vi "Aquire LMS Data.vi"(10 "LMS Information Cluster In":T2) -> (2 "LMS Information Cluster Out":T1)   [LabVIEW 2014]
uses:
  Hokuyo URG Series.lvlib
panel:
  in  "Number of Scans":dbl
  in  "Scan Interval":dbl
  in  "Encoding Width":u16(ring)=3 items=["2 Byte"=2, "3 Byte"=3]
  in  "Cluster Count":dbl=1.0
  in  "Start Point":dbl=-135.0
  in  "End Point":dbl=135.0
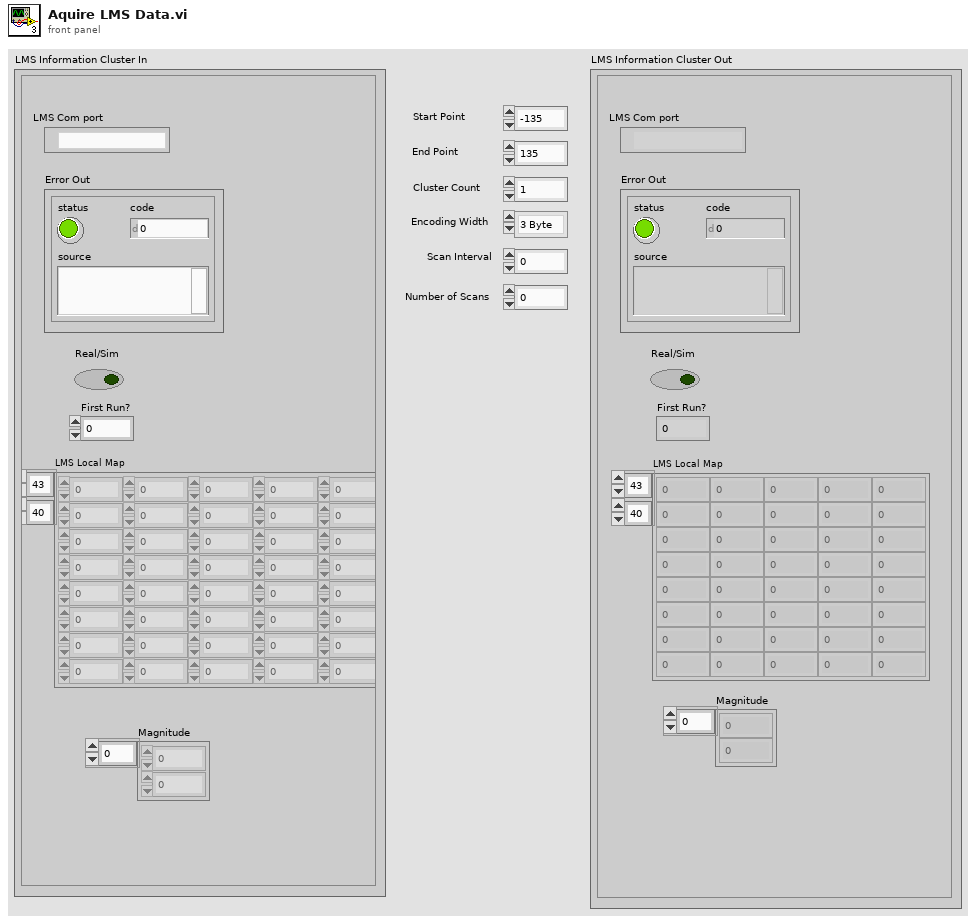
[diagram p1: front panel]
types:
  T1 = cluster{"LMS Com port":refnum<visa-resource-name>, "Error Out":errorcluster, "Real/Sim":bool, "First Run?":i32, "LMS Local Map ":dbl[][], "Magnitude":dbl[]}
  T2 = cluster{"LMS Com port":refnum<visa-resource-name>, "Error Out":errorcluster, "Real/Sim":bool, "First Run?":i32, "LMS Local Map ":i32[][], "Magnitude":dbl[]}
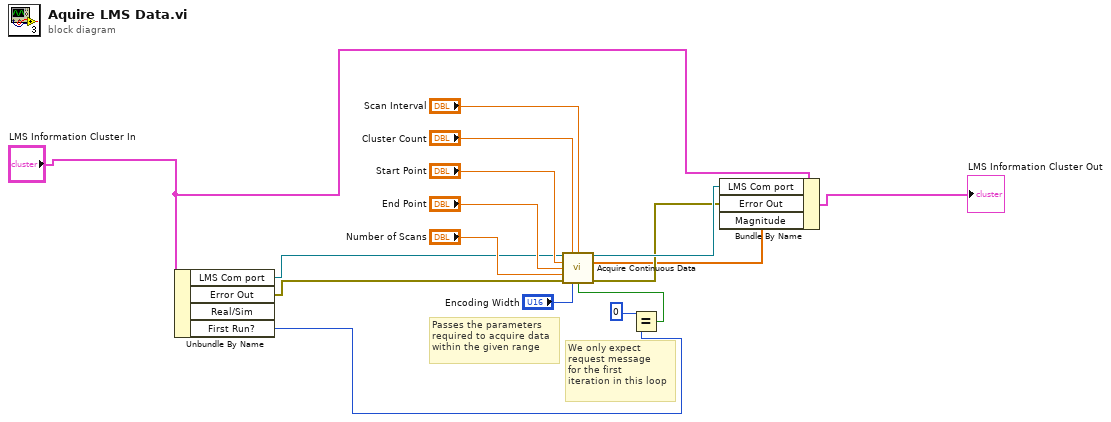
[diagram p0: block diagram]
diagram:
  # "We only expect\nrequest message\nfor the first\niteration in this loop"
  # "Passes the parameters\nrequired to acquire data\nwithin the given range"
  n1 = Unbundle By Name("LMS Information Cluster In") -> ("LMS Com port"=w8:refnum<visa-resource-name>, "Error Out"=w7:errorcluster, "First Run?"=w6:i32)  [unwired: 1 out]
  n2 = Equal?(x=0, y=w6) -> (x = y?=w9:bool)
  n3 = call "Acquire Continuous Data.vi"("VISA resource name"=w8, "Cluster Count (1)"="Cluster Count", "Scan Interval (1)"="Scan Interval", "Start Point (-120°)"="Start Point", "End Point (120°)"="End Point", "Number of Scans (0)"="Number of Scans", "error in (no error)"=w7, "Data Encoding Width (3 Byte)"="Encoding Width", "Enable Request Message (F:Disable)"=w9) -> ("VISA resource name out"=w4:refnum<visa-resource-name>, "Magnitude"=w2:dbl[], "error out"=w3:errorcluster)  [unwired: 1 in, 3 out]
  n4 = Bundle By Name(cluster="LMS Information Cluster In", "LMS Com port"=w4, "Error Out"=w3, "Magnitude"=w2) -> (→"LMS Information Cluster Out":T2)
